vi "nanocal -- nuclear schottky fit V8.vi"() -> ()   [LabVIEW 2021] (continued)
 \"τ22\" -> 0.000000000000   ,  \"τN1\" -> 0.000000000000   ,  \"τN2\" -> 0.000000000000   ,  \"σηlogτ1 \" -> 0.081363569031   ,  \"σηlogτS\" -> 0.000000046538   ,  \"σηlogτN\" -> 0.121425477475   ,  \"σlogτ1\" -> 11.127970233063   ,  \"σlogτS\" -> 0.000080214100   ,  \"σlogτN\" -> 8.138592608049   ,  \"σητ1\" -> 0.001314492921   ,  \"σητS \" -> 0.000000000280   ,  \"σητN\" -> 0.000000032203    |>   , \n\"IDS0593_220608_RAW_cal__sam_\" ->   <|    \"ζ\" -> 0.000000000000   ,  \"τ1\" -> 0.000000000000   ,  \"τS\" -> 0.000000000000   ,  \"τN\" -> 0.000000000000   ,  \"τC\" -> 0.000000000000   ,  \"κ0\" -> 0.000000000000   ,  \"mm1\" -> 0.000000000000   ,  \"mm2\" -> 0.000000000000   ,  \"mm3\" -> 0.000000000000   ,  \"T\" -> 5.700000000000   ,  \"B\" -> 2.000000000000   ,  \"θ\" -> 90.000000000000   ,  \"Reoff\" -> 0.000000000000   ,  \"Imoff\" -> 0.000000000000   ,  \"στ1\" -> 0.000000000000   ,  \"στS\" -> 0.000000000000   ,  \"στN\" -> 0.000000000000   ,  \"τ11 \" -> 0.000000000000   ,  \"τ12\" -> 0.000000000000   ,  \"τ22\" -> 0.000000000000   ,  \"τN1\" -> 0.000000000000   ,  \"τN2\" -> 0.000000000000   ,  \"σηlogτ1 \" -> 0.000000000000   ,  \"σηlogτS\" -> 0.000000000000   ,  \"σηlogτN\" -> 0.000000000000   ,  \"σlogτ1\" -> 0.000000000000   ,  \"σlogτS\" -> 0.000000000000   ,  \"σlogτN\" -> 0.000000000000   ,  \"σητ1\" -> 0.000000000000   ,  \"σητS \" -> 0.000000000000   ,  \"σητN\" -> 0.000000000000    |>   , \n\"IDS0595_220608_RAW_cal__ref_\" ->   <|    \"ζ\" -> 0.244875688813   ,  \"τ1\" -> 0.040857302003   ,  \"τS\" -> 0.046628683614   ,  \"τN\" -> 0.009593794520   ,  \"τC\" -> 0.000917891247   ,  \"κ0\" -> 0.000000000890   ,  \"mm1\" -> 0.000178281936   ,  \"mm2\" -> 0.029128430859   ,  \"mm3\" -> 0.082458476649   ,  \"T\" -> 0.200000000000   ,  \"B\" -> 4.000000000000   ,  \"θ\" -> 90.000000000000   ,  \"Reoff\" -> 0.000000000000   ,  \"Imoff\" -> 0.000000000000   ,  \"στ1\" -> 0.000204250954   ,  \"στS\" -> 0.000016140182   ,  \"στN\" -> 0.000025700358   ,  \"τ11 \" -> 0.000000000000   ,  \"τ12\" -> 0.000000000000   ,  \"τ22\" -> 0.000000000000   ,  \"τN1\" -> 0.000000000000   ,  \"τN2\" -> 0.000000000000   ,  \"σηlogτ1 \" -> 0.133588413120   ,  \"σηlogτS\" -> 0.001269402003   ,  \"σηlogτN\" -> 0.135197574519   ,  \"σlogτ1\" -> 0.004999129754   ,  \"σlogτS\" -> 0.000346142779   ,  \"σlogτN\" -> 0.002678852216   ,  \"σητ1\" -> 0.005458062139   ,  \"σητS \" -> 0.000059190544   ,  \"σητN\" -> 0.001297057749    |>   , \n\"IDS0595_220608_RAW_cal__sam_\" ->   <|    \"ζ\" -> 0.000000000000   ,  \"τ1\" -> 0.000000000000   ,  \"τS\" -> 0.000000000000   ,  \"τN\" -> 0.000000000000   ,  \"τC\" -> 0.000000000000   ,  \"κ0\" -> 0.000000000000   ,  \"mm1\" -> 0.000000000000   ,  \"mm2\" -> 0.000000000000   ,  \"mm3\" -> 0.000000000000   ,  \"T\" -> 0.200000000000   ,  \"B\" -> 4.000000000000   ,  \"θ\" -> 90.000000000000   ,  \"Reoff\" -> 0.000000000000   ,  \"Imoff\" -> 0.000000000000   ,  \"στ1\" -> 0.000000000000   ,  \"στS\" -> 0.000000000000   ,  \"στN\" -> 0.000000000000   ,  \"τ11 \" -> 0.000000000000   ,  \"τ12\" -> 0.000000000000   ,  \"τ22\" -> 0.000000000000   ,  \"τN1\" -> 0.000000000000   ,  \"τN2\" -> 0.000000000000   ,  \"σηlogτ1 \" -> 0.000000000000   ,  \"σηlogτS\" -> 0.000000000000   ,  \"σηlogτN\" -> 0.000000000000   ,  \"σlogτ1\" -> 0.000000000000   ,  \"σlogτS\" -> 0.000000000000   ,  \"σlogτN\" -> 0.000000000000   ,  \"σητ1\" -> 0.000000000000   ,  \"σητS \" -> 0.000000000000   ,  \"σητN\" -> 0.000000000000    |>   , \n\"IDS0596_220608_RAW_cal__ref_\" ->   <|    \"ζ\" -> 0.344647843466   ,  \"τ1\" -> 0.055962851231   ,  \"τS\" -> 0.054806527829   ,  \"τN\" -> 0.019330510227   ,  \"τC\" -> 0.000846071488   ,  \"κ0\" -> 0.000000000723   ,  \"mm1\" -> 0.000215013630   ,  \"mm2\" -> 0.034022445863   ,  \"mm3\" -> 0.122259671569   ,  \"T\" -> 0.170000000000   ,  \"B\" -> 4.000000000000   ,  \"θ\" -> 90.000000000000   ,  \"Reoff\" -> 0.000000000000   ,  \"Imoff\" -> 0.000000000000   ,  \"στ1\" -> 0.000271742026   ,  \"στS\" -> 0.000028779791   ,  \"στN\" -> 0.000052361049   ,  \"τ11 \" -> 0.000000000000   ,  \"τ12\" -> 0.000000000000   ,  \"τ22\" -> 0.000000000000   ,  \"τN1\" -> 0.000000000000   ,  \"τN2\" -> 0.000000000000   ,  \"σηlogτ1 \" -> 0.127696466200   ,  \"σηlogτS\" -> 0.001816681804   ,  \"σηlogτN\" -> 0.135107921466   ,  \"σlogτ1\" -> 0.004855757346   ,  \"σlogτS\" -> 0.000525116114   ,  \"σlogτN\" -> 0.002708725676   ,  \"σητ1\" -> 0.007146258341   ,  \"σητS \" -> 0.000099566022   ,  \"σητN\" -> 0.002611705058    |>   , \n\"IDS0596_220608_RAW_cal__sam_\" ->   <|    \"ζ\" -> 0.000000000000   ,  \"τ1\" -> 0.000000000000   ,  \"τS\" -> 0.000000000000   ,  \"τN\" -> 0.000000000000   ,  \"τC\" -> 0.000000000000   ,  \"κ0\" -> 0.000000000000   ,  \"mm1\" -> 0.000000000000   ,  \"mm2\" -> 0.000000000000   ,  \"mm3\" -> 0.000000000000   ,  \"T\" -> 0.170000000000   ,  \"B\" -> 4.000000000000   ,  \"θ\" -> 90.000000000000   ,  \"Reoff\" -> 0.000000000000   ,  \"Imoff\" -> 0.000000000000   ,  \"στ1\" -> 0.000000000000   ,  \"στS\" -> 0.000000000000   ,  \"στN\" -> 0.000000000000   ,  \"τ11 \" -> 0.000000000000   ,  \"τ12\" -> 0.000000000000   ,  \"τ22\" -> 0.000000000000   ,  \"τN1\" -> 0.000000000000   ,  \"τN2\" -> 0.000000000000   ,  \"σηlogτ1 \" -> 0.000000000000   ,  \"σηlogτS\" -> 0.000000000000   ,  \"σηlogτN\" -> 0.000000000000   ,  \"σlogτ1\" -> 0.000000000000   ,  \"σlogτS\" -> 0.000000000000   ,  \"σlogτN\" -> 0.000000000000   ,  \"σητ1\" -> 0.000000000000   ,  \"σητS \" -> 0.000000000000   ,  \"σητN\" -> 0.000000000000    |>   , \n\"IDS0597_220608_RAW_cal__ref_\" ->   <|    \"ζ\" -> 0.438135386554   ,  \"τ1\" -> 0.068308117245   ,  \"τS\" -> 0.065117760308   ,  \"τN\" -> 0.029655865549   ,  \"τC\" -> 0.000827290289   ,  \"κ0\" -> 0.000000000603   ,  \"mm1\" -> 0.000250492842   ,  \"mm2\" -> 0.038649413418   ,  \"mm3\" -> 0.166532806331   ,  \"T\" -> 0.150000000000   ,  \"B\" -> 4.000000000000   ,  \"θ\" -> 90.000000000000   ,  \"Reoff\" -> 0.000000000000   ,  \"Imoff\" -> 0.000000000000   ,  \"στ1\" -> 0.000386864233   ,  \"στS\" -> 0.000050730025   ,  \"στN\" -> 0.000093978346   ,  \"τ11 \" -> 0.000000000000   ,  \"τ12\" -> 0.000000000000   ,  \"τ22\" -> 0.000000000000   ,  \"τN1\" -> 0.000000000000   ,  \"τN2\" -> 0.000000000000   ,  \"σηlogτ1 \" -> 0.130185307771   ,  \"σηlogτS\" -> 0.002377860764   ,  \"σηlogτN\" -> 0.136705910950   ,  \"σlogτ1\" -> 0.005663517726   ,  \"σlogτS\" -> 0.000779050517   ,  \"σlogτN\" -> 0.003168963187   ,  \"σητ1\" -> 0.008892713267   ,  \"σητS \" -> 0.000154840967   ,  \"σητN\" -> 0.004054132115    |>   , \n\"IDS0597_220608_RAW_cal__sam_\" ->   <|    \"ζ\" -> 0.000000000000   ,  \"τ1\" -> 0.000000000000   ,  \"τS\" -> 0.000000000000   ,  \"τN\" -> 0.000000000000   ,  \"τC\" -> 0.000000000000   ,  \"κ0\" -> 0.000000000000   ,  \"mm1\" -> 0.000000000000   ,  \"mm2\" -> 0.000000000000   ,  \"mm3\" -> 0.000000000000   ,  \"T\" -> 0.150000000000   ,  \"B\" -> 4.000000000000   ,  \"θ\" -> 90.000000000000   ,  \"Reoff\" -> 0.000000000000   ,  \"Imoff\" -> 0.000000000000   ,  \"στ1\" -> 0.000000000000   ,  \"στS\" -> 0.000000000000   ,  \"στN\" -> 0.000000000000   ,  \"τ11 \" -> 0.000000000000   ,  \"τ12\" -> 0.000000000000   ,  \"τ22\" -> 0.000000000000   ,  \"τN1\" -> 0.000000000000   ,  \"τN2\" -> 0.000000000000   ,  \"σηlogτ1 \" -> 0.000000000000   ,  \"σηlogτS\" -> 0.000000000000   ,  \"σηlogτN\" -> 0.000000000000   ,  \"σlogτ1\" -> 0.000000000000   ,  \"σlogτS\" -> 0.000000000000   ,  \"σlogτN\" -> 0.000000000000   ,  \"σητ1\" -> 0.000000000000   ,  \"σητS \" -> 0.000000000000   ,  \"σητN\" -> 0.000000000000    |>   , \n\"IDS0598_220609_RAW_cal__ref_\" ->   <|    \"ζ\" -> 0.657739242664   ,  \"τ1\" -> 0.094390866023   ,  \"τS\" -> 0.092485939026   ,  \"τN\" -> 0.075235660574   ,  \"τC\" -> 0.000808280402   ,  \"κ0\" -> 0.000000000441   ,  \"mm1\" -> 0.000319678865   ,  \"mm2\" -> 0.044160231701   ,  \"mm3\" -> 0.328757913357   ,  \"T\" -> 0.120000000000   ,  \"B\" -> 4.000000000000   ,  \"θ\" -> 90.000000000000   ,  \"Reoff\" -> 0.000000000000   ,  \"Imoff\" -> 0.000000000000   ,  \"στ1\" -> 0.000620717106   ,  \"στS\" -> 0.000143661942   ,  \"στN\" -> 0.000275186110   ,  \"τ11 \" -> 0.000000000000   ,  \"τ12\" -> 0.000000000000   ,  \"τ22\" -> 0.000000000000   ,  \"τN1\" -> 0.000000000000   ,  \"τN2\" -> 0.000000000000   ,  \"σηlogτ1 \" -> 0.141859959037   ,  \"σηlogτS\" -> 0.004605254266   ,  \"σηlogτN\" -> 0.143938852633   ,  \"σlogτ1\" -> 0.006576029356   ,  \"σlogτS\" -> 0.001553338196   ,  \"σlogτN\" -> 0.003657655270   ,  \"σητ1\" -> 0.013390284387   ,  \"σητS \" -> 0.000425921265   ,  \"σητN\" -> 0.010829334660    |>   , \n\"IDS0598_220609_RAW_cal__sam_\" ->   <|    \"ζ\" -> 0.000000000000   ,  \"τ1\" -> 0.000000000000   ,  \"τS\" -> 0.000000000000   ,  \"τN\" -> 0.000000000000   ,  \"τC\" -> 0.000000000000   ,  \"κ0\" -> 0.000000000000   ,  \"mm1\" -> 0.000000000000   ,  \"mm2\" -> 0.000000000000   ,  \"mm3\" -> 0.000000000000   ,  \"T\" -> 0.120000000000   ,  \"B\" -> 4.000000000000   ,  \"θ\" -> 90.000000000000   ,  \"Reoff\" -> 0.000000000000   ,  \"Imoff\" -> 0.000000000000   ,  \"στ1\" -> 0.000000000000   ,  \"στS\" -> 0.000000000000   ,  \"στN\" -> 0.000000000000   ,  \"τ11 \" -> 0.000000000000   ,  \"τ12\" -> 0.000000000000   ,  \"τ22\" -> 0.000000000000   ,  \"τN1\" -> 0.000000000000   ,  \"τN2\" -> 0.000000000000   ,  \"σηlogτ1 \" -> 0.000000000000   ,  \"σηlogτS\" -> 0.000000000000   ,  \"σηlogτN\" -> 0.000000000000   ,  \"σlogτ1\" -> 0.000000000000   ,  \"σlogτS\" -> 0.000000000000   ,  \"σlogτN\" -> 0.000000000000   ,  \"σητ1\" -> 0.000000000000   ,  \"σητS \" -> 0.000000000000   ,  \"σητN\" -> 0.000000000000    |>   , \n\"IDS0599_220609_RAW_cal__ref_\" ->   <|    \"ζ\" -> 0.160640867986   ,  \"τ1\" -> 0.030730944542   ,  \"τS\" -> 0.038747882734   ,  \"τN\" -> 0.003719905451   ,  \"τC\" -> 0.000979240032   ,  \"κ0\" -> 0.000000001232   ,  \"mm1\" -> 0.000133029555   ,  \"mm2\" -> 0.025373328786   ,  \"mm3\" -> 0.055493676773   ,  \"T\" -> 0.250000000000   ,  \"B\" -> 4.000000000000   ,  \"θ\" -> 90.000000000000   ,  \"Reoff\" -> 0.000000000000   ,  \"Imoff\" -> 0.000000000000   ,  \"στ1\" -> 0.000234620158   ,  \"στS\" -> 0.000010118580   ,  \"στN\" -> 0.000014838249   ,  \"τ11 \" -> 0.000000000000   ,  \"τ12\" -> 0.000000000000   ,  \"τ22\" -> 0.000000000000   ,  \"τN1\" -> 0.000000000000   ,  \"τN2\" -> 0.000000000000   ,  \"σηlogτ1 \" -> 0.136644624286   ,  \"σηlogτS\" -> 0.000655650020   ,  \"σηlogτN\" -> 0.134783134887   ,  \"σlogτ1\" -> 0.007634654967   ,  \"σlogτS\" -> 0.000261138906   ,  \"σlogτN\" -> 0.003988877910   ,  \"σητ1\" -> 0.004199218371   ,  \"σητS \" -> 0.000025405050   ,  \"σητN\" -> 0.000501380518    |>   , \n\"IDS0599_220609_RAW_cal__sam_\" ->   <|    \"ζ\" -> 0.000000000000   ,  \"τ1\" -> 0.000000000000   ,  \"τS\" -> 0.000000000000   ,  \"τN\" -> 0.000000000000   ,  \"τC\" -> 0.000000000000   ,  \"κ0\" -> 0.000000000000   ,  \"mm1\" -> 0.000000000000   ,  \"mm2\" -> 0.000000000000   ,  \"mm3\" -> 0.000000000000   ,  \"T\" -> 0.250000000000   ,  \"B\" -> 4.000000000000   ,  \"θ\" -> 90.000000000000   ,  \"Reoff\" -> 0.000000000000   ,  \"Imoff\" -> 0.000000000000   ,  \"στ1\" -> 0.000000000000   ,  \"στS\" -> 0.000000000000   ,  \"στN\" -> 0.000000000000   ,  \"τ11 \" -> 0.000000000000   ,  \"τ12\" -> 0.000000000000   ,  \"τ22\" -> 0.000000000000   ,  \"τN1\" -> 0.000000000000   ,  \"τN2\" -> 0.000000000000   ,  \"σηlogτ1 \" -> 0.000000000000   ,  \"σηlogτS\" -> 0.000000000000   ,  \"σηlogτN\" -> 0.000000000000   ,  \"σlogτ1\" -> 0.000000000000   ,  \"σlogτS\" -> 0.000000000000   ,  \"σlogτN\" -> 0.000000000000   ,  \"σητ1\" -> 0.000000000000   ,  \"σητS \" -> 0.000000000000   ,  \"σητN\" -> 0.000000000000    |>   , \n\"IDS0601_220609_RAW_cal__ref_\" ->   <|    \"ζ\" -> 0.076065163691   ,  \"τ1\" -> 0.031218215846   ,  \"τS\" -> 0.032891504670   ,  \"τN\" -> 0.001274630230   ,  \"τC\" -> 0.001592613462   ,  \"κ0\" -> 0.000000001977   ,  \"mm1\" -> 0.000108046468   ,  \"mm2\" -> 0.027306090435   ,  \"mm3\" -> 0.042161679950   ,  \"T\" -> 0.360000000000   ,  \"B\" -> 4.000000000000   ,  \"θ\" -> 90.000000000000   ,  \"Reoff\" -> 0.000000000000   ,  \"Imoff\" -> 0.000000000000   ,  \"στ1\" -> 0.000358946293   ,  \"στS\" -> 0.000004673235   ,  \"στN\" -> 0.000008052665   ,  \"τ11 \" -> 0.000000000000   ,  \"τ12\" -> 0.000000000000   ,  \"τ22\" -> 0.000000000000   ,  \"τN1\" -> 0.000000000000   ,  \"τN2\" -> 0.000000000000   ,  \"σηlogτ1 \" -> 0.120490592225   ,  \"σηlogτS\" -> 0.000188213230   ,  \"σηlogτN\" -> 0.130970976261   ,  \"σlogτ1\" -> 0.011497975887   ,  \"σlogτS\" -> 0.000142080293   ,  \"σlogτN\" -> 0.006317648081   ,  \"σητ1\" -> 0.003761501315   ,  \"σητS \" -> 0.000006190616   ,  \"σητN\" -> 0.000166939566    |>   , \n\"IDS0601_220609_RAW_cal__sam_\" ->   <|    \"ζ\" -> 0.000000000000   ,  \"τ1\" -> 0.000000000000   ,  \"τS\" -> 0.000000000000   ,  \"τN\" -> 0.000000000000   ,  \"τC\" -> 0.000000000000   ,  \"κ0\" -> 0.000000000000   ,  \"mm1\" -> 0.000000000000   ,  \"mm2\" -> 0.000000000000   ,  \"mm3\" -> 0.000000000000   ,  \"T\" -> 0.360000000000   ,  \"B\" -> 4.000000000000   ,  \"θ\" -> 90.000000000000   ,  \"Reoff\" -> 0.000000000000   ,  \"Imoff\" -> 0.000000000000   ,  \"στ1\" -> 0.000000000000   ,  \"στS\" -> 0.000000000000   ,  \"στN\" -> 0.000000000000   ,  \"τ11 \" -> 0.000000000000   ,  \"τ12\" -> 0.000000000000   ,  \"τ22\" -> 0.000000000000   ,  \"τN1\" -> 0.000000000000   ,  \"τN2\" -> 0.000000000000   ,  \"σηlogτ1 \" -> 0.000000000000   ,  \"σηlogτS\" -> 0.000000000000   ,  \"σηlogτN\" -> 0.000000000000   ,  \"σlogτ1\" -> 0.000000000000   ,  \"σlogτS\" -> 0.000000000000   ,  \"σlogτN\" -> 0.000000000000   ,  \"σητ1\" -> 0.000000000000   ,  \"σητS \" -> 0.000000000000   ,  \"σητN\" -> 0.000000000000    |>   , \n\"IDS0602_220609_RAW_cal__ref_\" ->   <|    \"ζ\" -> 0.057533507223   ,  \"τ1\" -> 0.029396748260   ,  \"τS\" -> 0.031273780346   ,  \"τN\" -> 0.000872241596   ,  \"τC\" -> 0.001990785128   ,  \"κ0\" -> 0.000000002387   ,  \"mm1\" -> 0.000102455319   ,  \"mm2\" -> 0.026505841871   ,  \"mm3\" -> 0.038774731525   ,  \"T\" -> 0.420000000000   ,  \"B\" -> 4.000000000000   ,  \"θ\" -> 90.000000000000   ,  \"Reoff\" -> 0.000000000000   ,  \"Imoff\" -> 0.000000000000   ,  \"στ1\" -> 0.000352874051   ,  \"στS\" -> 0.000003364822   ,  \"στN\" -> 0.000005730274   ,  \"τ11 \" -> 0.000000000000   ,  \"τ12\" -> 0.000000000000   ,  \"τ22\" -> 0.000000000000   ,  \"τN1\" -> 0.000000000000   ,  \"τN2\" -> 0.000000000000   ,  \"σηlogτ1 \" -> 0.120950197398   ,  \"σηlogτS\" -> 0.000137548204   ,  \"σηlogτN\" -> 0.130993605381   ,  \"σlogτ1\" -> 0.012003846422   ,  \"σlogτS\" -> 0.000107592440   ,  \"σlogτN\" -> 0.006569595024   ,  \"σητ1\" -> 0.003555542505   ,  \"σητS \" -> 0.000004301652   ,  \"σητN\" -> 0.000114258071    |>   , \n\"IDS0602_220609_RAW_cal__sam_\" ->   <|    \"ζ\" -> 0.000000000000   ,  \"τ1\" -> 0.000000000000   ,  \"τS\" -> 0.000000000000   ,  \"τN\" -> 0.000000000000   ,  \"τC\" -> 0.000000000000   ,  \"κ0\" -> 0.000000000000   ,  \"mm1\" -> 0.000000000000   ,  \"mm2\" -> 0.000000000000   ,  \"mm3\" -> 0.000000000000   ,  \"T\" -> 0.420000000000   ,  \"B\" -> 4.000000000000   ,  \"θ\" -> 90.000000000000   ,  \"Reoff\" -> 0.000000000000   ,  \"Imoff\" -> 0.000000000000   ,  \"στ1\" -> 0.000000000000   ,  \"στS\" -> 0.000000000000   ,  \"στN\" -> 0.000000000000   ,  \"τ11 \" -> 0.000000000000   ,  \"τ12\" -> 0.000000000000   ,  \"τ22\" -> 0.000000000000   ,  \"τN1\" -> 0.000000000000   ,  \"τN2\" -> 0.000000000000   ,  \"σηlogτ1 \" -> 0.000000000000   ,  \"σηlogτS\" -> 0.000000000000   ,  \"σηlogτN\" -> 0.000000000000   ,  \"σlogτ1\" -> 0.000000000000   ,  \"σlogτS\" -> 0.000000000000   ,  \"σlogτN\" -> 0.000000000000   ,  \"σητ1\" -> 0.000000000000   ,  \"σητS \" -> 0.000000000000   ,  \"σητN\" -> 0.000000000000    |>   , \n\"IDS0603_220609_RAW_cal__ref_\" ->   <|    \"ζ\" -> 0.041831727936   ,  \"τ1\" -> 0.022173847352   ,  \"τS\" -> 0.030659717390   ,  \"τN\" -> 0.000376835050   ,  \"τC\" -> 0.002231201000   ,  \"κ0\" -> 0.000000003055   ,  \"mm1\" -> 0.000083944151   ,  \"mm2\" -> 0.021503279099   ,  \"mm3\" -> 0.035152690160   ,  \"T\" -> 0.520000000000   ,  \"B\" -> 4.000000000000   ,  \"θ\" -> 90.000000000000   ,  \"Reoff\" -> 0.000000000000   ,  \"Imoff\" -> 0.000000000000   ,  \"στ1\" -> 0.000311741441   ,  \"στS\" -> 0.000001974777   ,  \"στN\" -> 0.000002711407   ,  \"τ11 \" -> 0.000000000000   ,  \"τ12\" -> 0.000000000000   ,  \"τ22\" -> 0.000000000000   ,  \"τN1\" -> 0.000000000000   ,  \"τN2\" -> 0.000000000000   ,  \"σηlogτ1 \" -> 0.139454796721   ,  \"σηlogτS\" -> 0.000091254795   ,  \"σηlogτN\" -> 0.134491686536   ,  \"σlogτ1\" -> 0.014058969391   ,  \"σlogτS\" -> 0.000064409512   ,  \"σlogτN\" -> 0.007195210096   ,  \"σητ1\" -> 0.003092249375   ,  \"σητS \" -> 0.000002797846   ,  \"σητN\" -> 0.000050681181    |>   , \n\"IDS0603_220609_RAW_cal__sam_\" ->   <|    \"ζ\" -> 0.000000000000   ,  \"τ1\" -> 0.000000000000   ,  \"τS\" -> 0.000000000000   ,  \"τN\" -> 0.000000000000   ,  \"τC\" -> 0.000000000000   ,  \"κ0\" -> 0.000000000000   ,  \"mm1\" -> 0.000000000000   ,  \"mm2\" -> 0.000000000000   ,  \"mm3\" -> 0.000000000000   ,  \"T\" -> 0.520000000000   ,  \"B\" -> 4.000000000000   ,  \"θ\" -> 90.000000000000   ,  \"Reoff\" -> 0.000000000000   ,  \"Imoff\" -> 0.000000000000   ,  \"στ1\" -> 0.000000000000   ,  \"στS\" -> 0.000000000000   ,  \"στN\" -> 0.000000000000   ,  \"τ11 \" -> 0.000000000000   ,  \"τ12\" -> 0.000000000000   ,  \"τ22\" -> 0.000000000000   ,  \"τN1\" -> 0.000000000000   ,  \"τN2\" -> 0.000000000000   ,  \"σηlogτ1 \" -> 0.000000000000   ,  \"σηlogτS\" -> 0.000000000000   ,  \"σηlogτN\" -> 0.000000000000   ,  \"σlogτ1\" -> 0.000000000000   ,  \"σlogτS\" -> 0.000000000000   ,  \"σlogτN\" -> 0.000000000000   ,  \"σητ1\" -> 0.000000000000   ,  \"σητS \" -> 0.000000000000   ,  \"σητN\" -> 0.000000000000    |>   , \n\"IDS0604_220609_RAW_cal__ref_\" ->   <|    \"ζ\" -> 0.032626148375   ,  \"τ1\" -> 0.016295992277   ,  \"τS\" -> 0.030913389463   ,  \"τN\" -> 0.000240237020   ,  \"τC\" -> 0.002587979957   ,  \"κ0\" -> 0.000000003764   ,  \"mm1\" -> 0.000075802373   ,  \"mm2\" -> 0.016078766991   ,  \"mm3\" -> 0.034899452194   ,  \"T\" -> 0.620000000000   ,  \"B\" -> 4.000000000000   ,  \"θ\" -> 90.000000000000   ,  \"Reoff\" -> 0.000000000000   ,  \"Imoff\" -> 0.000000000000   ,  \"στ1\" -> 0.000253503530   ,  \"στS\" -> 0.000001618253   ,  \"στN\" -> 0.000001840465   ,  \"τ11 \" -> 0.000000000000   ,  \"τ12\" -> 0.000000000000   ,  \"τ22\" -> 0.000000000000   ,  \"τN1\" -> 0.000000000000   ,  \"τN2\" -> 0.000000000000   ,  \"σηlogτ1 \" -> 0.168215723146   ,  \"σηlogτS\" -> 0.000092448124   ,  \"σηlogτN\" -> 0.139242705944   ,  \"σlogτ1\" -> 0.015556188633   ,  \"σlogτS\" -> 0.000052347952   ,  \"σlogτN\" -> 0.007661039077   ,  \"σητ1\" -> 0.002741242125   ,  \"σητS \" -> 0.000002857885   ,  \"σητN\" -> 0.000033451253    |>   , \n\"IDS0604_220609_RAW_cal__sam_\" ->   <|    \"ζ\" -> 0.000000000000   ,  \"τ1\" -> 0.000000000000   ,  \"τS\" -> 0.000000000000   ,  \"τN\" -> 0.000000000000   ,  \"τC\" -> 0.000000000000   ,  \"κ0\" -> 0.000000000000   ,  \"mm1\" -> 0.000000000000   ,  \"mm2\" -> 0.000000000000   ,  \"mm3\" -> 0.000000000000   ,  \"T\" -> 0.620000000000   ,  \"B\" -> 4.000000000000   ,  \"θ\" -> 90.000000000000   ,  \"Reoff\" -> 0.000000000000   ,  \"Imoff\" -> 0.000000000000   ,  \"στ1\" -> 0.000000000000   ,  \"στS\" -> 0.000000000000   ,  \"στN\" -> 0.000000000000   ,  \"τ11 \" -> 0.000000000000   ,  \"τ12\" -> 0.000000000000   ,  \"τ22\" -> 0.000000000000   ,  \"τN1\" -> 0.000000000000   ,  \"τN2\" -> 0.000000000000   ,  \"σηlogτ1 \" -> 0.000000000000   ,  \"σηlogτS\" -> 0.000000000000   ,  \"σηlogτN\" -> 0.000000000000   ,  \"σlogτ1\" -> 0.000000000000   ,  \"σlogτS\" -> 0.000000000000   ,  \"σlogτN\" -> 0.000000000000   ,  \"σητ1\" -> 0.000000000000   ,  \"σητS \" -> 0.000000000000   ,  \"σητN\" -> 0.000000000000    |>   , \n\"IDS0605_220609_RAW_cal__ref_\" ->   <|    \"ζ\" -> 0.023859329163   ,  \"τ1\" -> 0.019602952610   ,  \"τS\" -> 0.033018385867   ,  \"τN\" -> 0.000076995064   ,  \"τC\" -> 0.003545555695   ,  \"κ0\" -> 0.000000005104   ,  \"mm1\" -> 0.000074930617   ,  \"mm2\" -> 0.019516360911   ,  \"mm3\" -> 0.037442231294   ,  \"T\" -> 0.820000000000   ,  \"B\" -> 4.000000000000   ,  \"θ\" -> 90.000000000000   ,  \"Reoff\" -> 0.000000000000   ,  \"Imoff\" -> 0.000000000000   ,  \"στ1\" -> 0.001189137867   ,  \"στS\" -> 0.000001934551   ,  \"στN\" -> 0.000002314405   ,  \"τ11 \" -> 0.000000000000   ,  \"τ12\" -> 0.000000000000   ,  \"τ22\" -> 0.000000000000   ,  \"τN1\" -> 0.000000000000   ,  \"τN2\" -> 0.000000000000   ,  \"σηlogτ1 \" -> 0.157953519412   ,  \"σηlogτS\" -> 0.000023861164   ,  \"σηlogτN\" -> 0.137571798355   ,  \"σlogτ1\" -> 0.060661161144   ,  \"σlogτS\" -> 0.000058590114   ,  \"σlogτN\" -> 0.030059136097   ,  \"σητ1\" -> 0.003096355356   ,  \"σητS \" -> 0.000000787857   ,  \"σητN\" -> 0.000010592349    |>   , \n\"IDS0605_220609_RAW_cal__sam_\" ->   <|    \"ζ\" -> 0.000000000000   ,  \"τ1\" -> 0.000000000000   ,  \"τS\" -> 0.000000000000   ,  \"τN\" -> 0.000000000000   ,  \"τC\" -> 0.000000000000   ,  \"κ0\" -> 0.000000000000   ,  \"mm1\" -> 0.000000000000   ,  \"mm2\" -> 0.000000000000   ,  \"mm3\" -> 0.000000000000   ,  \"T\" -> 0.820000000000   ,  \"B\" -> 4.000000000000   ,  \"θ\" -> 90.000000000000   ,  \"Reoff\" -> 0.000000000000   ,  \"Imoff\" -> 0.000000000000   ,  \"στ1\" -> 0.000000000000   ,  \"στS\" -> 0.000000000000   ,  \"στN\" -> 0.000000000000   ,  \"τ11 \" -> 0.000000000000   ,  \"τ12\" -> 0.000000000000   ,  \"τ22\" -> 0.000000000000   ,  \"τN1\" -> 0.000000000000   ,  \"τN2\" -> 0.000000000000   ,  \"σηlogτ1 \" -> 0.000000000000   ,  \"σηlogτS\" -> 0.000000000000   ,  \"σηlogτN\" -> 0.000000000000   ,  \"σlogτ1\" -> 0.000000000000   ,  \"σlogτS\" -> 0.000000000000   ,  \"σlogτN\" -> 0.000000000000   ,  \"σητ1\" -> 0.000000000000   ,  \"σητS \" -> 0.000000000000   ,  \"σητN\" -> 0.000000000000    |>   , \n\"IDS0606_220609_RAW_cal__ref_\" ->   <|    \"ζ\" -> 0.021435159495   ,  \"τ1\" -> 0.026151503947   ,  \"τS\" -> 0.039003049453   ,  \"τN\" -> 0.000032134248   ,  \"τC\" -> 0.001875690429   ,  \"κ0\" -> 0.000000007011   ,  \"mm1\" -> 0.000037626031   ,  \"mm2\" -> 0.026096531119   ,  \"mm3\" -> 0.041764946316   ,  \"T\" -> 1.100000000000   ,  \"B\" -> 4.000000000000   ,  \"θ\" -> 90.000000000000   ,  \"Reoff\" -> -840816.326530613004   ,  \"Imoff\" -> 0.000000000000   ,  \"στ1\" -> 0.182357772529   ,  \"στS\" -> 0.000092921705   ,  \"στN\" -> 0.090781245007   ,  \"τ11 \" -> 0.000000000000   ,  \"τ12\" -> 0.000000000000   ,  \"τ22\" -> 0.000000000000   ,  \"τN1\" -> 0.000000000000   ,  \"τN2\" -> 0.000000000000   ,  \"σηlogτ1 \" -> 0.000000000000   ,  \"σηlogτS\" -> 0.000000000000   ,  \"σηlogτN\" -> 0.000000000000   ,  \"σlogτ1\" -> 0.000000000000   ,  \"σlogτS\" -> 0.000000000000   ,  \"σlogτN\" -> 0.000000000000   ,  \"σητ1\" -> 0.000000000000   ,  \"σητS \" -> 0.000000000000   ,  \"σητN\" -> 0.000000000000    |>   , \n\"IDS0606_220609_RAW_cal__sam_\" ->   <|    \"ζ\" -> 0.000000000000   ,  \"τ1\" -> 0.000000000000   ,  \"τS\" -> 0.000000000000   ,  \"τN\" -> 0.000000000000   ,  \"τC\" -> 0.000000000000   ,  \"κ0\" -> 0.000000000000   ,  \"mm1\" -> 0.000000000000   ,  \"mm2\" -> 0.000000000000   ,  \"mm3\" -> 0.000000000000   ,  \"T\" -> 1.100000000000   ,  \"B\" -> 4.000000000000   ,  \"θ\" -> 90.000000000000   ,  \"Reoff\" -> 0.000000000000   ,  \"Imoff\" -> 0.000000000000   ,  \"στ1\" -> 0.000000000000   ,  \"στS\" -> 0.000000000000   ,  \"στN\" -> 0.000000000000   ,  \"τ11 \" -> 0.000000000000   ,  \"τ12\" -> 0.000000000000   ,  \"τ22\" -> 0.000000000000   ,  \"τN1\" -> 0.000000000000   ,  \"τN2\" -> 0.000000000000   ,  \"σηlogτ1 \" -> 0.000000000000   ,  \"σηlogτS\" -> 0.000000000000   ,  \"σηlogτN\" -> 0.000000000000   ,  \"σlogτ1\" -> 0.000000000000   ,  \"σlogτS\" -> 0.000000000000   ,  \"σlogτN\" -> 0.000000000000   ,  \"σητ1\" -> 0.000000000000   ,  \"σητS \" -> 0.000000000000   ,  \"σητN\" -> 0.000000000000    |>   , \n\"IDS0607_220609_RAW_cal__ref_\" ->   <|    \"ζ\" -> 0.019275949161   ,  \"τ1\" -> 0.024231785659   ,  \"τS\" -> 0.015186052952   ,  \"τN\" -> 0.000011847591   ,  \"τC\" -> 0.002181793311   ,  \"κ0\" -> 0.000000010412   ,  \"mm1\" -> 0.000036237774   ,  \"mm2\" -> 0.017592345864   ,  \"mm3\" -> 0.024275849834   ,  \"T\" -> 1.600000000000   ,  \"B\" -> 4.000000000000   ,  \"θ\" -> 90.000000000000   ,  \"Reoff\" -> -583673.469387755030   ,  \"Imoff\" -> 0.000000000000   ,  \"στ1\" -> 0.299468636941   ,  \"στS\" -> 0.000091809023   ,  \"στN\" -> 0.139501640547   ,  \"τ11 \" -> 0.000000000000   ,  \"τ12\" -> 0.000000000000   ,  \"τ22\" -> 0.000000000000   ,  \"τN1\" -> 0.000000000000   ,  \"τN2\" -> 0.000000000000   ,  \"σηlogτ1 \" -> 0.000000000000   ,  \"σηlogτS\" -> 0.000000000000   ,  \"σηlogτN\" -> 0.000000000000   ,  \"σlogτ1\" -> 0.000000000000   ,  \"σlogτS\" -> 0.000000000000   ,  \"σlogτN\" -> 0.000000000000   ,  \"σητ1\" -> 0.000000000000   ,  \"σητS \" -> 0.000000000000   ,  \"σητN\" -> 0.000000000000    |>   , \n\"IDS0607_220609_RAW_cal__sam_\" ->   <|    \"ζ\" -> 0.000000000000   ,  \"τ1\" -> 0.000000000000   ,  \"τS\" -> 0.000000000000   ,  \"τN\" -> 0.000000000000   ,  \"τC\" -> 0.000000000000   ,  \"κ0\" -> 0.000000000000   ,  \"mm1\" -> 0.000000000000   ,  \"mm2\" -> 0.000000000000   ,  \"mm3\" -> 0.000000000000   ,  \"T\" -> 1.600000000000   ,  \"B\" -> 4.000000000000   ,  \"θ\" -> 90.000000000000   ,  \"Reoff\" -> 0.000000000000   ,  \"Imoff\" -> 0.000000000000   ,  \"στ1\" -> 0.000000000000   ,  \"στS\" -> 0.000000000000   ,  \"στN\" -> 0.000000000000   ,  \"τ11 \" -> 0.000000000000   ,  \"τ12\" -> 0.000000000000   ,  \"τ22\" -> 0.000000000000   ,  \"τN1\" -> 0.000000000000   ,  \"τN2\" -> 0.000000000000   ,  \"σηlogτ1 \" -> 0.000000000000   ,  \"σηlogτS\" -> 0.000000000000   ,  \"σηlogτN\" -> 0.000000000000   ,  \"σlogτ1\" -> 0.000000000000   ,  \"σlogτS\" -> 0.000000000000   ,  \"σlogτN\" -> 0.000000000000   ,  \"σητ1\" -> 0.000000000000   ,  \"σητS \" -> 0.000000000000   ,  \"σητN\" -> 0.000000000000    |>   , \n\"IDS0608_220610_RAW_cal__ref_\" ->   <|    \"ζ\" -> 0.016336803082   ,  \"τ1\" -> 0.018850208513   ,  \"τS\" -> 0.013770021313   ,  \"τN\" -> 0.000006308743   ,  \"τC\" -> 0.002013144857   ,  \"κ0\" -> 0.000000012633   ,  \"mm1\" -> 0.000028340387   ,  \"mm2\" -> 0.015944607726   ,  \"mm3\" -> 0.018891796505   ,  \"T\" -> 1.900000000000   ,  \"B\" -> 4.000000000000   ,  \"θ\" -> 90.000000000000   ,  \"Reoff\" -> -306122.448979591834   ,  \"Imoff\" -> 0.000000000000   ,  \"στ1\" -> 0.600607467529   ,  \"στS\" -> 0.000120470426   ,  \"στN\" -> 0.265461721995   ,  \"τ11 \" -> 0.000000000000   ,  \"τ12\" -> 0.000000000000   ,  \"τ22\" -> 0.000000000000   ,  \"τN1\" -> 0.000000000000   ,  \"τN2\" -> 0.000000000000   ,  \"σηlogτ1 \" -> 0.000000000000   ,  \"σηlogτS\" -> 0.000000000000   ,  \"σηlogτN\" -> 0.000000000000   ,  \"σlogτ1\" -> 0.000000000000   ,  \"σlogτS\" -> 0.000000000000   ,  \"σlogτN\" -> 0.000000000000   ,  \"σητ1\" -> 0.000000000000   ,  \"σητS \" -> 0.000000000000   ,  \"σητN\" -> 0.000000000000    |>   , \n\"IDS0608_220610_RAW_cal__sam_\" ->   <|    \"ζ\" -> 0.000000000000   ,  \"τ1\" -> 0.000000000000   ,  \"τS\" -> 0.000000000000   ,  \"τN\" -> 0.000000000000   ,  \"τC\" -> 0.000000000000   ,  \"κ0\" -> 0.000000000000   ,  \"mm1\" -> 0.000000000000   ,  \"mm2\" -> 0.000000000000   ,  \"mm3\" -> 0.000000000000   ,  \"T\" -> 1.900000000000   ,  \"B\" -> 4.000000000000   ,  \"θ\" -> 90.000000000000   ,  \"Reoff\" -> 0.000000000000   ,  \"Imoff\" -> 0.000000000000   ,  \"στ1\" -> 0.000000000000   ,  \"στS\" -> 0.000000000000   ,  \"στN\" -> 0.000000000000   ,  \"τ11 \" -> 0.000000000000   ,  \"τ12\" -> 0.000000000000   ,  \"τ22\" -> 0.000000000000   ,  \"τN1\" -> 0.000000000000   ,  \"τN2\" -> 0.000000000000   ,  \"σηlogτ1 \" -> 0.000000000000   ,  \"σηlogτS\" -> 0.000000000000   ,  \"σηlogτN\" -> 0.000000000000   ,  \"σlogτ1\" -> 0.000000000000   ,  \"σlogτS\" -> 0.000000000000   ,  \"σlogτN\" -> 0.000000000000   ,  \"σητ1\" -> 0.000000000000   ,  \"σητS \" -> 0.000000000000   ,  \"σητN\" -> 0.000000000000    |>   , \n\"IDS0609_220610_RAW_cal__ref_\" ->   <|    \"ζ\" -> 0.016902895564   ,  \"τ1\" -> 0.016875930626   ,  \"τS\" -> 0.009655247253   ,  \"τN\" -> 0.000001449904   ,  \"τC\" -> 0.002468410143   ,  \"κ0\" -> 0.000000022390   ,  \"mm1\" -> 0.000032874904   ,  \"mm2\" -> 0.012250082224   ,  \"mm3\" -> 0.016881306941   ,  \"T\" -> 3.100000000000   ,  \"B\" -> 4.000000000000   ,  \"θ\" -> 90.000000000000   ,  \"Reoff\" -> -175510.204081632662   ,  \"Imoff\" -> 0.000000000000   ,  \"στ1\" -> 3.649351876038   ,  \"στS\" -> 0.000215288637   ,  \"στN\" -> 1.699153814821   ,  \"τ11 \" -> 0.000000000000   ,  \"τ12\" -> 0.000000000000   ,  \"τ22\" -> 0.000000000000   ,  \"τN1\" -> 0.000000000000   ,  \"τN2\" -> 0.000000000000   ,  \"σηlogτ1 \" -> 0.000000000000   ,  \"σηlogτS\" -> 0.000000000000   ,  \"σηlogτN\" -> 0.000000000000   ,  \"σlogτ1\" -> 0.000000000000   ,  \"σlogτS\" -> 0.000000000000   ,  \"σlogτN\" -> 0.000000000000   ,  \"σητ1\" -> 0.000000000000   ,  \"σητS \" -> 0.000000000000   ,  \"σητN\" -> 0.000000000000    |>   , \n\"IDS0609_220610_RAW_cal__sam_\" ->   <|    \"ζ\" -> 0.000000000000   ,  \"τ1\" -> 0.000000000000   ,  \"τS\" -> 0.000000000000   ,  \"τN\" -> 0.000000000000   ,  \"τC\" -> 0.000000000000   ,  \"κ0\" -> 0.000000000000   ,  \"mm1\" -> 0.000000000000   ,  \"mm2\" -> 0.000000000000   ,  \"mm3\" -> 0.000000000000   ,  \"T\" -> 3.100000000000   ,  \"B\" -> 4.000000000000   ,  \"θ\" -> 90.000000000000   ,  \"Reoff\" -> 0.000000000000   ,  \"Imoff\" -> 0.000000000000   ,  \"στ1\" -> 0.000000000000   ,  \"στS\" -> 0.000000000000   ,  \"στN\" -> 0.000000000000   ,  \"τ11 \" -> 0.000000000000   ,  \"τ12\" -> 0.000000000000   ,  \"τ22\" -> 0.000000000000   ,  \"τN1\" -> 0.000000000000   ,  \"τN2\" -> 0.000000000000   ,  \"σηlogτ1 \" -> 0.000000000000   ,  \"σηlogτS\" -> 0.000000000000   ,  \"σηlogτN\" -> 0.000000000000   ,  \"σlogτ1\" -> 0.000000000000   ,  \"σlogτS\" -> 0.000000000000   ,  \"σlogτN\" -> 0.000000000000   ,  \"σητ1\" -> 0.000000000000   ,  \"σητS \" -> 0.000000000000   ,  \"σητN\" -> 0.000000000000    |>   , \n\"IDS0610_220610_RAW_cal__ref_\" ->   <|    \"ζ\" -> 0.018202138450   ,  \"τ1\" -> 0.014600581263   ,  \"τS\" -> 0.005986495902   ,  \"τN\" -> 0.000000194501   ,  \"τC\" -> 0.002004933118   ,  \"κ0\" -> 0.000000055137   ,  \"mm1\" -> 0.000027060886   ,  \"mm2\" -> 0.008073090494   ,  \"mm3\" -> 0.014601023972   ,  \"T\" -> 5.700000000000   ,  \"B\" -> 4.000000000000   ,  \"θ\" -> 90.000000000000   ,  \"Reoff\" -> -61224.489795918343   ,  \"Imoff\" -> 0.000000000000   ,  \"στ1\" -> 47.935064380633   ,  \"στS\" -> 0.000496948445   ,  \"στN\" -> 25.454668996980   ,  \"τ11 \" -> 0.000000000000   ,  \"τ12\" -> 0.000000000000   ,  \"τ22\" -> 0.000000000000   ,  \"τN1\" -> 0.000000000000   ,  \"τN2\" -> 0.000000000000   ,  \"σηlogτ1 \" -> 0.000000000000   ,  \"σηlogτS\" -> 0.000000000000   ,  \"σηlogτN\" -> 0.000000000000   ,  \"σlogτ1\" -> 0.000000000000   ,  \"σlogτS\" -> 0.000000000000   ,  \"σlogτN\" -> 0.000000000000   ,  \"σητ1\" -> 0.000000000000   ,  \"σητS \" -> 0.000000000000   ,  \"σητN\" -> 0.000000000000    |>   , \n\"IDS0610_220610_RAW_cal__sam_\" ->   <|    \"ζ\" -> 0.000000000000   ,  \"τ1\" -> 0.000000000000   ,  \"τS\" -> 0.000000000000   ,  \"τN\" -> 0.000000000000   ,  \"τC\" -> 0.000000000000   ,  \"κ0\" -> 0.000000000000   ,  \"mm1\" -> 0.000000000000   ,  \"mm2\" -> 0.000000000000   ,  \"mm3\" -> 0.000000000000   ,  \"T\" -> 5.700000000000   ,  \"B\" -> 4.000000000000   ,  \"θ\" -> 90.000000000000   ,  \"Reoff\" -> 0.000000000000   ,  \"Imoff\" -> 0.000000000000   ,  \"στ1\" -> 0.000000000000   ,  \"στS\" -> 0.000000000000   ,  \"στN\" -> 0.000000000000   ,  \"τ11 \" -> 0.000000000000   ,  \"τ12\" -> 0.000000000000   ,  \"τ22\" -> 0.000000000000   ,  \"τN1\" -> 0.000000000000   ,  \"τN2\" -> 0.000000000000   ,  \"σηlogτ1 \" -> 0.000000000000   ,  \"σηlogτS\" -> 0.000000000000   ,  \"σηlogτN\" -> 0.000000000000   ,  \"σlogτ1\" -> 0.000000000000   ,  \"σlogτS\" -> 0.000000000000   ,  \"σlogτN\" -> 0.000000000000   ,  \"σητ1\" -> 0.000000000000   ,  \"σητS \" -> 0.000000000000   ,  \"σητN\" -> 0.000000000000    |>   , \n\"IDS0612_220610_RAW_cal__ref_\" ->   <|    \"ζ\" -> 0.027806171987   ,  \"τ1\" -> 0.017638558844   ,  \"τS\" -> 0.022454693159   ,  \"τN\" -> 0.000161041319   ,  \"τC\" -> 0.002790453039   ,  \"κ0\" -> 0.000000005094   ,  \"mm1\" -> 0.000067525595   ,  \"mm2\" -> 0.017301806666   ,  \"mm3\" -> 0.026304271103   ,  \"T\" -> 0.820000000000   ,  \"B\" -> 5.000000000000   ,  \"θ\" -> 90.000000000000   ,  \"Reoff\" -> 0.000000000000   ,  \"Imoff\" -> 0.000000000000   ,  \"στ1\" -> 0.000450123313   ,  \"στS\" -> 0.000001495593   ,  \"στN\" -> 0.000002123028   ,  \"τ11 \" -> 0.000000000000   ,  \"τ12\" -> 0.000000000000   ,  \"τ22\" -> 0.000000000000   ,  \"τN1\" -> 0.000000000000   ,  \"τN2\" -> 0.000000000000   ,  \"σηlogτ1 \" -> 0.135604423187   ,  \"σηlogτS\" -> 0.000049481364   ,  \"σηlogτN\" -> 0.133726108983   ,  \"σlogτ1\" -> 0.025519279466   ,  \"σlogτS\" -> 0.000066604901   ,  \"σlogτN\" -> 0.013183126504   ,  \"σητ1\" -> 0.002391866598   ,  \"σητS \" -> 0.000001111089   ,  \"σητN\" -> 0.000021535429    |>   , \n\"IDS0612_220610_RAW_cal__sam_\" ->   <|    \"ζ\" -> 0.000000000000   ,  \"τ1\" -> 0.000000000000   ,  \"τS\" -> 0.000000000000   ,  \"τN\" -> 0.000000000000   ,  \"τC\" -> 0.000000000000   ,  \"κ0\" -> 0.000000000000   ,  \"mm1\" -> 0.000000000000   ,  \"mm2\" -> 0.000000000000   ,  \"mm3\" -> 0.000000000000   ,  \"T\" -> 0.820000000000   ,  \"B\" -> 5.000000000000   ,  \"θ\" -> 90.000000000000   ,  \"Reoff\" -> 0.000000000000   ,  \"Imoff\" -> 0.000000000000   ,  \"στ1\" -> 0.000000000000   ,  \"στS\" -> 0.000000000000   ,  \"στN\" -> 0.000000000000   ,  \"τ11 \" -> 0.000000000000   ,  \"τ12\" -> 0.000000000000   ,  \"τ22\" -> 0.000000000000   ,  \"τN1\" -> 0.000000000000   ,  \"τN2\" -> 0.000000000000   ,  \"σηlogτ1 \" -> 0.000000000000   ,  \"σηlogτS\" -> 0.000000000000   ,  \"σηlogτN\" -> 0.000000000000   ,  \"σlogτ1\" -> 0.000000000000   ,  \"σlogτS\" -> 0.000000000000   ,  \"σlogτN\" -> 0.000000000000   ,  \"σητ1\" -> 0.000000000000   ,  \"σητS \" -> 0.000000000000   ,  \"σητN\" -> 0.000000000000    |>   , \n\"IDS0613_220610_RAW_cal__ref_\" ->   <|    \"ζ\" -> 0.023917075048   ,  \"τ1\" -> 0.017613265802   ,  \"τS\" -> 0.018183300032   ,  \"τN\" -> 0.000057867909   ,  \"τC\" -> 0.002629507092   ,  \"κ0\" -> 0.000000007146   ,  \"mm1\" -> 0.000053956897   ,  \"mm2\" -> 0.017346246578   ,  \"mm3\" -> 0.021520012742   ,  \"T\" -> 1.120000000000   ,  \"B\" -> 5.000000000000   ,  \"θ\" -> 90.000000000000   ,  \"Reoff\" -> 0.000000000000   ,  \"Imoff\" -> 0.000000000000   ,  \"στ1\" -> 0.001474274081   ,  \"στS\" -> 0.000001579241   ,  \"στN\" -> 0.000002631422   ,  \"τ11 \" -> 0.000000000000   ,  \"τ12\" -> 0.000000000000   ,  \"τ22\" -> 0.000000000000   ,  \"τN1\" -> 0.000000000000   ,  \"τN2\" -> 0.000000000000   ,  \"σηlogτ1 \" -> 0.121751267744   ,  \"σηlogτS\" -> 0.000016109653   ,  \"σηlogτN\" -> 0.131002454305   ,  \"σlogτ1\" -> 0.083702482984   ,  \"σlogτS\" -> 0.000086851191   ,  \"σlogτN\" -> 0.045472911920   ,  \"σητ1\" -> 0.002144437441   ,  \"σητS \" -> 0.000000292927   ,  \"σητN\" -> 0.000007580838    |>   , \n\"IDS0613_220610_RAW_cal__sam_\" ->   <|    \"ζ\" -> 0.000000000000   ,  \"τ1\" -> 0.000000000000   ,  \"τS\" -> 0.000000000000   ,  \"τN\" -> 0.000000000000   ,  \"τC\" -> 0.000000000000   ,  \"κ0\" -> 0.000000000000   ,  \"mm1\" -> 0.000000000000   ,  \"mm2\" -> 0.000000000000   ,  \"mm3\" -> 0.000000000000   ,  \"T\" -> 1.120000000000   ,  \"B\" -> 5.000000000000   ,  \"θ\" -> 90.000000000000   ,  \"Reoff\" -> 0.000000000000   ,  \"Imoff\" -> 0.000000000000   ,  \"στ1\" -> 0.000000000000   ,  \"στS\" -> 0.000000000000   ,  \"στN\" -> 0.000000000000   ,  \"τ11 \" -> 0.000000000000   ,  \"τ12\" -> 0.000000000000   ,  \"τ22\" -> 0.000000000000   ,  \"τN1\" -> 0.000000000000   ,  \"τN2\" -> 0.000000000000   ,  \"σηlogτ1 \" -> 0.000000000000   ,  \"σηlogτS\" -> 0.000000000000   ,  \"σηlogτN\" -> 0.000000000000   ,  \"σlogτ1\" -> 0.000000000000   ,  \"σlogτS\" -> 0.000000000000   ,  \"σlogτN\" -> 0.000000000000   ,  \"σητ1\" -> 0.000000000000   ,  \"σητS \" -> 0.000000000000   ,  \"σητN\" -> 0.000000000000    |>   , \n\"IDS0614_220610_RAW_cal__ref_\" ->   <|    \"ζ\" -> 0.017909358082   ,  \"τ1\" -> 0.017480687226   ,  \"τS\" -> 0.012860329043   ,  \"τN\" -> 0.000018141436   ,  \"τC\" -> 0.003015067786   ,  \"κ0\" -> 0.000000012573   ,  \"mm1\" -> 0.000043233082   ,  \"mm2\" -> 0.015879465115   ,  \"mm3\" -> 0.017682172433   ,  \"T\" -> 1.900000000000   ,  \"B\" -> 5.000000000000   ,  \"θ\" -> 90.000000000000   ,  \"Reoff\" -> 0.000000000000   ,  \"Imoff\" -> 0.000000000000   ,  \"στ1\" -> 0.004241418912   ,  \"στS\" -> 0.000001205375   ,  \"στN\" -> 0.000002608933   ,  \"τ11 \" -> 0.000000000000   ,  \"τ12\" -> 0.000000000000   ,  \"τ22\" -> 0.000000000000   ,  \"τN1\" -> 0.000000000000   ,  \"τN2\" -> 0.000000000000   ,  \"σηlogτ1 \" -> 0.106069153141   ,  \"σηlogτS\" -> 0.000004568851   ,  \"σηlogτN\" -> 0.127617076550   ,  \"σlogτ1\" -> 0.242634563361   ,  \"σlogτS\" -> 0.000093728182   ,  \"σlogτN\" -> 0.143810713084   ,  \"σητ1\" -> 0.001854161690   ,  \"σητS \" -> 0.000000058757   ,  \"σητN\" -> 0.000002315157    |>   , \n\"IDS0614_220610_RAW_cal__sam_\" ->   <|    \"ζ\" -> 0.000000000000   ,  \"τ1\" -> 0.000000000000   ,  \"τS\" -> 0.000000000000   ,  \"τN\" -> 0.000000000000   ,  \"τC\" -> 0.000000000000   ,  \"κ0\" -> 0.000000000000   ,  \"mm1\" -> 0.000000000000   ,  \"mm2\" -> 0.000000000000   ,  \"mm3\" -> 0.000000000000   ,  \"T\" -> 1.900000000000   ,  \"B\" -> 5.000000000000   ,  \"θ\" -> 90.000000000000   ,  \"Reoff\" -> 0.000000000000   ,  \"Imoff\" -> 0.000000000000   ,  \"στ1\" -> 0.000000000000   ,  \"στS\" -> 0.000000000000   ,  \"στN\" -> 0.000000000000   ,  \"τ11 \" -> 0.000000000000   ,  \"τ12\" -> 0.000000000000   ,  \"τ22\" -> 0.000000000000   ,  \"τN1\" -> 0.000000000000   ,  \"τN2\" -> 0.000000000000   ,  \"σηlogτ1 \" -> 0.000000000000   ,  \"σηlogτS\" -> 0.000000000000   ,  \"σηlogτN\" -> 0.000000000000   ,  \"σlogτ1\" -> 0.000000000000   ,  \"σlogτS\" -> 0.000000000000   ,  \"σlogτN\" -> 0.000000000000   ,  \"σητ1\" -> 0.000000000000   ,  \"σητS \" -> 0.000000000000   ,  \"σητN\" -> 0.000000000000    |>   , \n\"IDS0615_220610_RAW_cal__ref_\" ->   <|    \"ζ\" -> 0.018184973350   ,  \"τ1\" -> 0.017408880913   ,  \"τS\" -> 0.009354983655   ,  \"τN\" -> 0.000004961796   ,  \"τC\" -> 0.002778499813   ,  \"κ0\" -> 0.000000022360   ,  \"mm1\" -> 0.000038538615   ,  \"mm2\" -> 0.012253069450   ,  \"mm3\" -> 0.017425928470   ,  \"T\" -> 3.100000000000   ,  \"B\" -> 5.000000000000   ,  \"θ\" -> 90.000000000000   ,  \"Reoff\" -> 0.000000000000   ,  \"Imoff\" -> 0.000000000000   ,  \"στ1\" -> 0.013841696755   ,  \"στS\" -> 0.000000886855   ,  \"στN\" -> 0.000002562855   ,  \"τ11 \" -> 0.000000000000   ,  \"τ12\" -> 0.000000000000   ,  \"τ22\" -> 0.000000000000   ,  \"τN1\" -> 0.000000000000   ,  \"τN2\" -> 0.000000000000   ,  \"σηlogτ1 \" -> 0.093950564075   ,  \"σηlogτS\" -> 0.000001087799   ,  \"σηlogτN\" -> 0.124728717422   ,  \"σlogτ1\" -> 0.795093999659   ,  \"σlogτS\" -> 0.000094800269   ,  \"σlogτN\" -> 0.516517527893   ,  \"σητ1\" -> 0.001635574182   ,  \"σητS \" -> 0.000000010176   ,  \"σητN\" -> 0.000000618878    |>   , \n\"IDS0615_220610_RAW_cal__sam_\" ->   <|    \"ζ\" -> 0.000000000000   ,  \"τ1\" -> 0.000000000000   ,  \"τS\" -> 0.000000000000   ,  \"τN\" -> 0.000000000000   ,  \"τC\" -> 0.000000000000   ,  \"κ0\" -> 0.000000000000   ,  \"mm1\" -> 0.000000000000   ,  \"mm2\" -> 0.000000000000   ,  \"mm3\" -> 0.000000000000   ,  \"T\" -> 3.100000000000   ,  \"B\" -> 5.000000000000   ,  \"θ\" -> 90.000000000000   ,  
